vi "dynamicfindway.vi"(4 "new_x":dbl, 6 "new_angle":dbl, 8 "angles":dbl[](array[numeric]), 9 "new_y":dbl, 10 "distances":dbl[](array[numeric]), 11 "Numeric":i32) -> (0 "preferredSteer":dbl, 1 "angleGoal":dbl, 2 "w_right":dbl, 3 "w_left":dbl)   [LabVIEW 2015]
uses:
  <vilib>/imath/engines/lvmath2/RunTimeEngine/IndexReplace/NIMS V(S)=S.vi
  <instcachedir>/0/NIMS V(S)=S_9916D32195284AEB9D40BA9A64F3B0C5.lvgen/NIMS V(S)=S_9916D32195284AEB9D40BA9A64F3B0C5_000.vi
  <vilib>/imathl/engines/lvmath/Functions/Error Handling/Create Error.vi
  <vilib>/imath/engines/lvmath2/RunTimeEngine/IndexRead/NIMS V(S).vi
  <instcachedir>/0/NIMS V(S)_0488751826AF41519A22953C041130DC.lvgen/NIMS V(S)_0488751826AF41519A22953C041130DC_000.vi
  <vilib>/imath/engines/lvmath2/RunTimeEngine/BuiltInFunctions/max/2 inputs/NIMS_max(RG,RG)-no size check.vi
  <instcachedir>/0/NIMS_max(RG,RG)-no size check_F871939977644B7683C1350DCCAD7557.lvgen/NIMS_max(RG,RG)-no size check_F871939977644B7683C1350DCCAD7557_000.vi
  <vilib>/imath/engines/lvmath2/RunTimeEngine/BuiltInFunctions/atan2/NIMS_atan2.vi
  <instcachedir>/0/NIMS_atan2_A91AA4A7D42247EDBE8F76DB99AF04A4.lvgen/NIMS_atan2_A91AA4A7D42247EDBE8F76DB99AF04A4_000.vi
  <vilib>/imath/engines/lvmath2/RunTimeEngine/ArithmeticOperatorToken/NIMS_ArithmeticOperator_power(S).vi
  <instcachedir>/0/NIMS_ArithmeticOperator_power(S)_DFB67823F1414E5097C86E39787D8CA8.lvgen/NIMS_ArithmeticOperator_power(S)_DFB67823F1414E5097C86E39787D8CA8_014.vi
  <vilib>/imath/engines/lvmath2/RunTimeEngine/ErrorHandling/NIMS_Create Error From Enums.vi
  <instcachedir>/0/NIMS_ArithmeticOperator_power(S)_DFB67823F1414E5097C86E39787D8CA8.lvgen/NIMS_ArithmeticOperator_power(S)_DFB67823F1414E5097C86E39787D8CA8_009.vi
  <vilib>/imath/engines/lvmath2/RunTimeEngine/BuiltInFunctions/max/1 input/NIMS_max(CV).vi
  <instcachedir>/0/NIMS_max(CV)_A85366AFBDD24459900A7FDE15250013.lvgen/NIMS_max(CV)_A85366AFBDD24459900A7FDE15250013_000.vi
  <instcachedir>/0/NIMS V(S)_0488751826AF41519A22953C041130DC.lvgen/NIMS V(S)_0488751826AF41519A22953C041130DC_003.vi
  <instcachedir>/0/NIMS_atan2_A91AA4A7D42247EDBE8F76DB99AF04A4.lvgen/NIMS_atan2_A91AA4A7D42247EDBE8F76DB99AF04A4_001.vi
  <vilib>/imath/engines/lvmath2/RunTimeEngine/CommandStatement/MC_CommandStatement_break.vi
  <vilib>/imath/engines/lvmath2/RunTimeEngine/CommandStatement/NIMS_CommandStatement_MaskErr.vi
  <vilib>/imath/engines/lvmath2/RunTimeEngine/VariableToken/NIMS_VariableToken_CondDefined.vi
  <instcachedir>/0/NIMS_VariableToken_CondDefined_FE30D0A1BFB24F098D41DEBABFE96BE1.lvgen/NIMS_VariableToken_CondDefined_FE30D0A1BFB24F098D41DEBABFE96BE1_004.vi
  <vilib>/imath/engines/lvmath2/RunTimeEngine/NodeEndStatement/NIMS_NodeEndStatement_Output.vi
  <instcachedir>/0/NIMS_NodeEndStatement_Output_53EC0D466D134D7ABD903AC30B43404B.lvgen/NIMS_NodeEndStatement_Output_53EC0D466D134D7ABD903AC30B43404B_001.vi
  <vilib>/imath/engines/lvmath2/RunTimeEngine/ErrorHandling/NIMS_Finalize Error.vi
panel:
  out "new_x 2":dbl
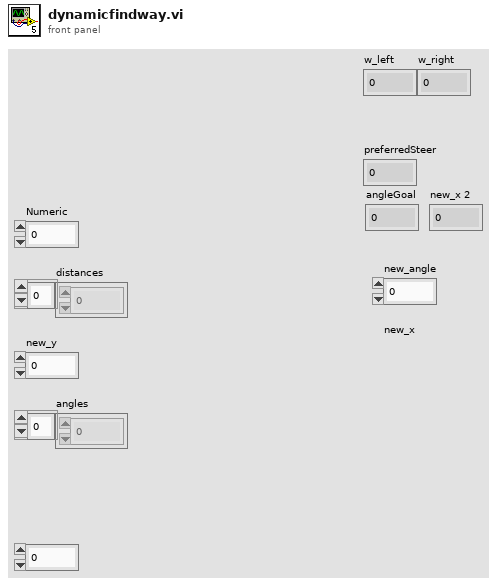
[diagram p1: front panel]
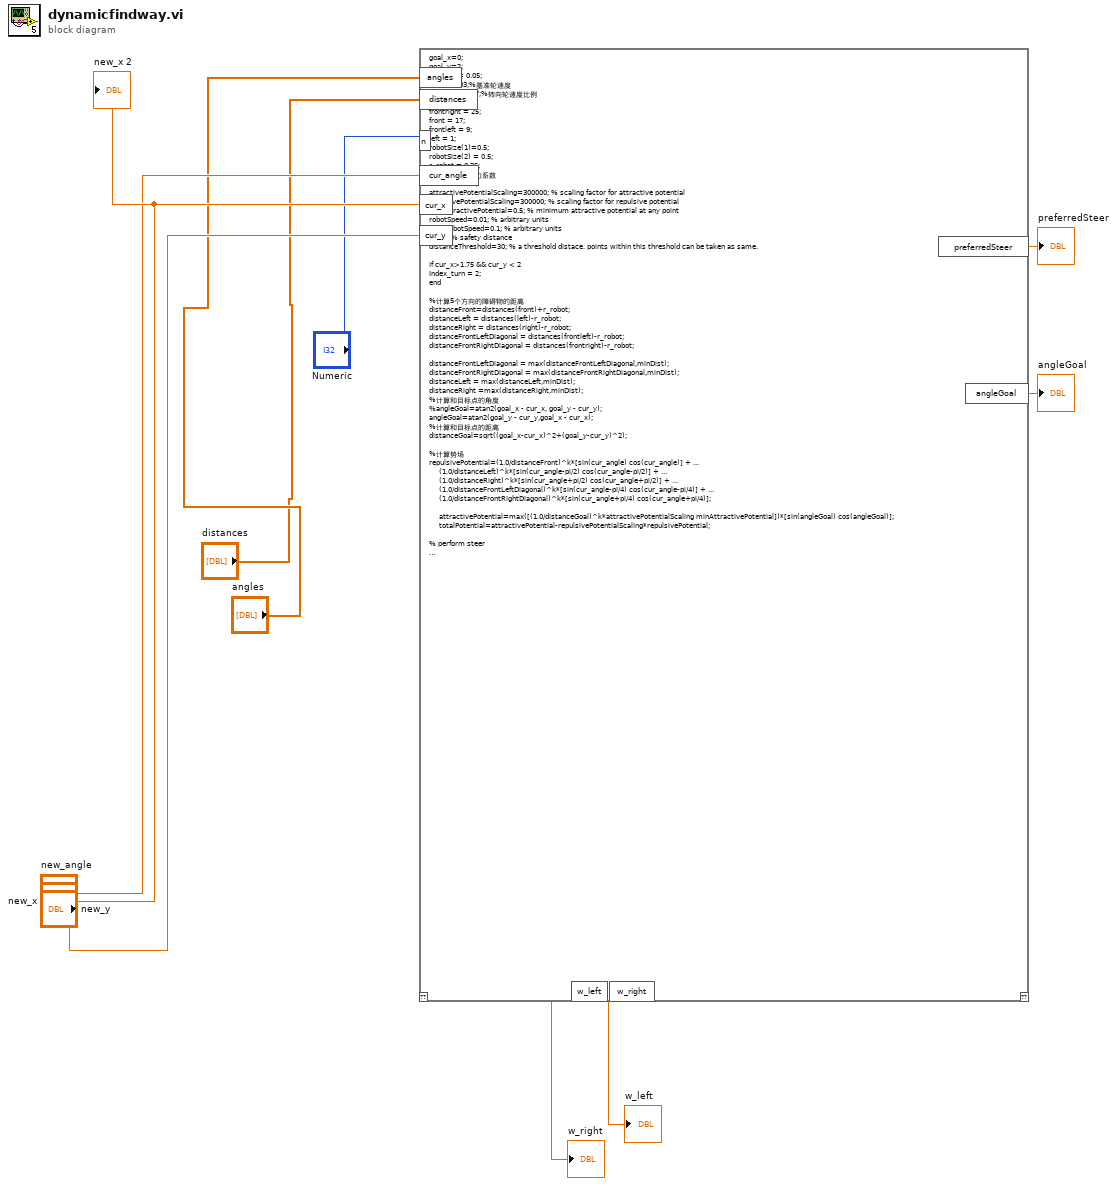
[diagram p0: block diagram]
diagram:
  n1 = mathscript code="goal_x=0;\ngoal_y=2;\nr_wheel = 0.05;\nVref = 0.03;%基准轮速度\nIndex_turn = 7;%转向轮速度比例\nright = 33;\nfrontright = 25;\nfront = 17;\nfrontleft = 9;\nleft = 1;\nrobotSize(1)=0.5;\nrobotSize(2) = 0.5;\nr_robot = 0.25;\nk = 1.25; %斥力系数\nminDist=0.03;\nattractivePotentialScaling=300000; % scaling factor for attractive potential\nrepulsivePotentialScaling=300000; % scaling factor for repulsive potential\nminAttractivePotential=0.5; % minimum attractive potential at any point\nrobotSpeed=0.01; % arbitrary units \nmaxRobotSpeed=0.1; % arbitrary units \nS=14; % safety distance\ndistanceThreshold=30; % a threshold distace. points within this threshold can be taken as same. \n\nif cur_x>1.75 && cur_y < 2\nIndex_turn = 2;\nend\n\n%计算5个方向的障碍物的距离\ndistanceFront=distances(front)+r_robot;\ndistanceLeft = distances(left)-r_robot;\ndistanceRight = distances(right)-r_robot;\ndistanceFrontLeftDiagonal = distances(frontleft)-r_robot;\ndistanceFrontRightDiagonal = distances(frontright)-r_robot;\n\ndistanceFrontLeftDiagonal = max(distanceFrontLeftDiagonal,minDist);\ndistanceFrontRightDiagonal = max(distanceFrontRightDiagonal,minDist);\ndistanceLeft = max(distanceLeft,minDist);\ndistanceRight =max(distanceRight,minDist);\n%计算和目标点的角度\n%angleGoal=atan2(goal_x - cur_x, goal_y - cur_y);\nangleGoal=atan2(goal_y - cur_y,goal_x - cur_x);\n%计算和目标点的距离\ndistanceGoal=sqrt((goal_x-cur_x)^2+(goal_y-cur_y)^2);\n\n%计算势场\nrepulsivePotential=(1.0/distanceFront)^k*[sin(cur_angle) cos(cur_angle)] + ...\n     (1.0/distanceLeft)^k*[sin(cur_angle-pi/2) cos(cur_angle-pi/2)] + ...\n     (1.0/distanceRight)^k*[sin(cur_angle+pi/2) cos(cur_angle+pi/2)] + ...\n     (1.0/distanceFrontLeftDiagonal)^k*[sin(cur_angle-pi/4) cos(cur_angle-pi/4)] + ...\n     (1.0/distanceFrontRightDiagonal)^k*[sin(cur_angle+pi/4) cos(cur_angle+pi/4)];\n     \n     attractivePotential=max([(1.0/distanceGoal)^k*attractivePotentialScaling minAttractivePotential])*[sin(angleGoal) cos(angleGoal)];\n     totalPotential=attractivePotential-repulsivePotentialScaling*repulsivePotential;\n\n% perform steer\n     preferredSteer = atan2(robotSpeed*sin(cur_angle)+totalPotential(1),robotSpeed*cos(cur_angle)+totalPotential(2))-cur_angle;\n     while preferredSteer>pi, preferredSteer=preferredSteer-2*pi; end % check to get the angle between -pi and pi\n     while preferredSteer<-pi, preferredSteer=preferredSteer+2*pi; end % check to get the angle between -pi and pi\n%      preferredSteer=min([maxTurn preferredSteer]);\n%      preferredSteer=max([-maxTurn preferredSteer]);\n%      currentDirection=currentDirection+preferredSteer;\n%      \n%      % setting the speed based on vehicle acceleration and speed limits. the vehicle cannot move backwards.\n%      preferredSpeed=sqrt(sum((robotSpeed*[sin(currentDirection) cos(currentDirection)] + totalPotential).^2));\n%      preferredSpeed=min([robotSpeed+maxAcceleration preferredSpeed]);\n%      robotSpeed=max([robotSpeed-maxAcceleration preferredSpeed]);\n%      robotSpeed=min([robotSpeed maxRobotSpeed]);\n% %      robotSpeed=max([robotSpeed 0]);\n    if preferredSteer>0   %需要左转\n        Vleft = Vref;\n        Vright = Vleft*Index_turn;\nend\n    if preferredSteer ==0\n        Vleft = Vref;\n         Vright = Vref;\n    end\nif preferredSteer<0\n        Vright = Vref;\n        Vleft = Vright*Index_turn;\n    end\n    \nw_right = Vright/r_wheel;\nw_left = Vleft/r_wheel;"("n"="Numeric", "distances"="distances", "angles"="angles", "cur_angle"="new_angle", "cur_x"="new_x", "cur_y"="new_y") -> ("w_left"=→"w_left":dbl, "w_right"=→"w_right":dbl, "preferredSteer"=→"preferredSteer":dbl, "angleGoal"=→"angleGoal":dbl)  [unwired: 1 in, 1 out]
  "new_x 2" <- "new_x"
